vi "Calculate Line Points.vi"(7 "Iterations":i32=10000, 9 "error in (no error)":errorcluster, 11 "Points":T1[](array[typedef])) -> (1 "error out":errorcluster, 2 "Y":dbl[](array[numeric]), 3 "X":dbl[](array[numeric]))   [LabVIEW 2019, in "Tool Path.lvclass"]
uses:
  Tool Path.lvclass
  Parse/PathCommands/Point.ctl
  Parse/PathCommands/PathCommands.lvclass
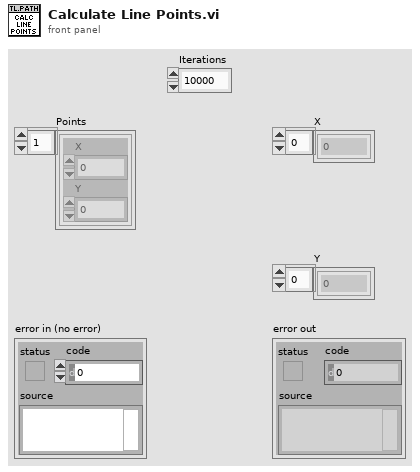
[diagram p1: front panel]
types:
  T1 = typedef "PathCommands.lvclass/Point.ctl" = cluster{"X":dbl, "Y":dbl}
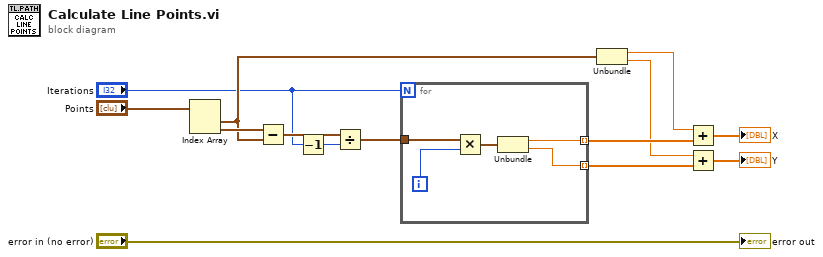
[diagram p0: block diagram]
diagram:
  n1 = Index Array(array="Points") -> (element #1=w10:T1, element #2=w13:T1)  [unwired: 2 in]
  n2 = Subtract(x=w13, y=w10) -> (x-y=w12:T1)
  n3 = Decrement(x="Iterations") -> (x-1=w2:i32)
  n4 = Divide(x=w12, y=w2) -> (x/y=w11:T1)
  n5 = for {
    N: "Iterations" -> [_]
    tunnel: w11 -> [w18]
    tunnel: [w15] -> w8 mode=indexing
    tunnel: [w16] -> w6 mode=indexing
    i -> [w19]
    n6 = Multiply(x=w18, y=w19) -> (x*y=w17:T1)
    n7 = Unbundle(w17) -> ("X"=w15:dbl, "Y"=w16:dbl)
  }
  n8 = Unbundle(w10) -> ("X"=w9:dbl, "Y"=w4:dbl)
  n9 = Add(x=w9, y=w8) -> (x+y=→"X":dbl[])
  n10 = Add(x=w4, y=w6) -> (x+y=→"Y":dbl[])
  "error out" <- "error in (no error)"
